vi "Main Tclk.vi"() -> ()   [LabVIEW 2018] (continued)
      n253 = property on="13nA Condenser (V)" class="DigNum (strict)"("Visible"=w181) -> ()  [unwired: 2 in, 2 out]
      n254 = local write "Status message"("standby" ("Status message")) -> ()
      n255 = local write "SEM Options"(w283) -> ()
      n256 = And(x=w164, y=w163) -> (x .and. y?=w162:bool)
      n257 = local write "Reheat completed"(w99) -> ()
      n258 = property on="Status Tabs" class="TabCtl (strict)"() -> ("Pages"=w189:refnum<vi>[])  [unwired: 2 in, 2 out]
      n259 = local write "Unfreeze"(w99) -> ()
      n260 = local write "Scan xn"(w99) -> ()
      n261 = Square Root(x=sgl 2.0 ("t")) -> (sqrt(x)=w104:sgl)
      n262 = local write "Milling para"(w301) -> ()
      n263 = property on="27nA Condenser (V)" class="DigNum (strict)"("Visible"=w181) -> ()  [unwired: 2 in, 2 out]
      n264 = property on="Reheat Output" class="Clust (strict)"("Visible"=w188) -> ()  [unwired: 2 in, 2 out]
      n265 = property on="Turn off FIB gun" class="Bool (strict)"("Visible"=w101) -> ()  [unwired: 2 in, 2 out]
      n266 = property on="Suppressor (V)" class="DigNum (strict)"("Visible"=TRUE) -> ()  [unwired: 2 in, 2 out]
      n267 = Divide(x=w105, y=w104) -> (x/y=w106:sgl)
      n268 = Index Array(array=w189, index=T11."HV Data" ("Status Tabs")) -> (element=w190:refnum<vi>)
      n269 = Select(t=w105, s=w162, f=w106) -> (s? t:f=w161:sgl)
      "X full scale (V)" <- w161
      n270 = local read "File Information"() -> (w286:T31)
      n271 = property class="DAQmx Device"("Active Device"=w248) -> (error out=w242:errorcluster, "AI.PhysicalChans"=w247:tag[])  [unwired: 2 in, 1 out]
      "Logging Channels" <- w247
      n272 = property class="Page"(reference=w190, "PageEnb"=w127) -> ()  [unwired: 1 in, 2 out]
      n273 = shared-variable ".\\Zeiss Library.lvlib\\X full scale (V)"(w161) -> ()  [unwired: 1 in, 1 out]
      n274 = property on="Open FIB gun valve" class="Bool (strict)"("Visible"=w101) -> ()  [unwired: 2 in, 2 out]
      n275 = property on="Image Tabs" class="TabCtl (strict)"() -> ("Pages"=w129:refnum<vi>[])  [unwired: 2 in, 2 out]
      n276 = Bundle By Name(cluster=w286, "File path"=path "E:/Images", "Save recipe"=w110, "Load recipe"=w110) -> (w285:T31)
      n277 = property on="Cursor Z (V)" class="DigNum (strict)"("Visible"=w110) -> ()  [unwired: 2 in, 2 out]
      n278 = Unbundle By Name(w242) -> ("status"=w241:bool)
      n279 = Array Size(array="Parameter Names") -> (size(s)=w244:i32)
      n280 = shared-variable ".\\Zeiss Library.lvlib\\Upload flags path"("D:\\UploadFlags" ("string")) -> ()  [unwired: 1 in, 1 out]
      n281 = property on="FIB Gun Valve Status" class="Str"("Visible"=w101) -> ()  [unwired: 2 in, 2 out]
      n282 = Array Subset(array=w247, length=w244) -> (w246:tag[])  [unwired: 1 in]
      n283 = Index Array(array=w129, index=T37."FIB HV Data" ("Image Tabs")) -> (element=w128:refnum<vi>)
      n284 = Build Path(base path=w113, name or relative path="Email Log") -> (appended path=w197:path)
      "Email Log Files" <- w197
      n285 = Build Path(base path=w113, name or relative path="FIB HV DataLog") -> (appended path=w201:path)
      "FIB HV DataLog Files" <- w201
      n286 = Build Path(base path=w113, name or relative path="SEM HV DataLog") -> (appended path=w152:path)
      "SEM HV DataLog Files" <- w152
      n287 = Build Path(base path=w113, name or relative path="Current DataLog") -> (appended path=w149:path)
      "Current DataLog Files" <- w149
      n288 = Build Path(base path=w113, name or relative path="FIB Reheat Log") -> (appended path=w179:path)
      "FIB Reheat Log Files" <- w179
      n289 = Build Path(base path=w113, name or relative path="Re-engage") -> (appended path=w115:path)
      "Re-engage Files" <- w115
      n290 = Build Path(base path=w113, name or relative path="FIB Probes.csv") -> (appended path=w116:path)
      n291 = Build Path(base path=w113, name or relative path="Last FIB milling snapshot.xml") -> (appended path=→"Last milling snapshot":path)
      n292 = Build Path(base path=w113, name or relative path="Last FIB recipe.csv") -> (appended path=→"Last FIB recipe":path)
      n293 = Build Path(base path=w113, name or relative path="Last FIB image.png") -> (appended path=→"Last FIB image":path)
      n294 = Build Path(base path=w113, name or relative path="Last FIB zoom pre image.png") -> (appended path=→"Last FIB zoom pre image":path)
      n295 = Build Path(base path=w113, name or relative path="Last DetA LM image.png") -> (appended path=→"Last Det A Low Mag":path)
      n296 = Build Path(base path=w113, name or relative path="Last DetB LM image.png") -> (appended path=→"Last Det B Low Mag":path)
      n297 = Build Path(base path=w113, name or relative path="Email alert recipients.txt") -> (appended path=w208:path)
      "Email recipents file" <- w208
      n298 = local write "File Information"(w285) -> ()
      n299 = property class="Page"(reference=w128, "PageEnb"=w127) -> ()  [unwired: 1 in, 2 out]
      n300 = property on="FIB Milling Objective (V)" class="DigNum (strict)"("Visible"=w101) -> ()  [unwired: 2 in, 2 out]
      n301 = property on="FIB Milling Probe" class="CmbBox"("Visible"=w101) -> ()  [unwired: 2 in, 2 out]
      n302 = Path To String(path=w113) -> (string=w114:string)
      n303 = File/Directory Info(path=w197) -> (path out=w194:path, error out=w196:errorcluster)  [unwired: 1 in, 5 out]
      n304 = File/Directory Info(path=w201) -> (path out=w204:path, error out=w202:errorcluster)  [unwired: 1 in, 5 out]
      n305 = File/Directory Info(path=w152) -> (path out=w153:path, error out=w155:errorcluster)  [unwired: 1 in, 5 out]
      n306 = File/Directory Info(path=w149) -> (path out=w148:path, error out=w146:errorcluster)  [unwired: 1 in, 5 out]
      n307 = File/Directory Info(path=w179) -> (path out=w176:path, error out=w178:errorcluster)  [unwired: 1 in, 5 out]
      n308 = File/Directory Info(path=w113) -> (path out=w237:path, error out=w239:errorcluster)  [unwired: 1 in, 5 out]
      n309 = File/Directory Info(path=w115) -> (path out=w218:path, error out=w216:errorcluster)  [unwired: 1 in, 5 out]
      n310 = call-poly <vilib>:"Read Delimited Spreadsheet.vi"("file path (dialog if empty)"=w116, "delimiter (\\t)"="," ("delimiter (\\t)")) -> ("all rows"=w94:string[][])  [unwired: 8 in, 5 out]
      n311 = call <vilib>:"DAQmx Flatten Channel String.vi"("names in"=w246) -> ("names out"=→"Active logging channels":string)  [unwired: 13 in, 1 out]
      n312 = shared-variable ".\\Zeiss Library.lvlib\\3D FIB-SEM Files Path"(w114) -> ()  [unwired: 1 in, 1 out]
      n313 = File/Directory Info(path=w208) -> (path out=w205:path, error out=w207:errorcluster)  [unwired: 1 in, 5 out]
      n314 = Unbundle By Name(w196) -> ("status"=w195:bool)
      n315 = Unbundle By Name(w202) -> ("status"=w203:bool)
      n316 = Unbundle By Name(w178) -> ("status"=w177:bool)
      n317 = Unbundle By Name(w216) -> ("status"=w217:bool)
      n318 = Array Size(array=w94) -> (size(s)=w122:i32[])
      n319 = Unbundle By Name(w155) -> ("status"=w154:bool)
      n320 = Unbundle By Name(w146) -> ("status"=w147:bool)
      n321 = Unbundle By Name(w239) -> ("status"=w238:bool)
      n322 = property on="Min FIB probe" class="Bool (strict)"("Visible"=w101) -> ()  [unwired: 2 in, 2 out]
      n323 = property on="Save Probe Table" class="Bool (strict)"("Visible"=w101) -> ()  [unwired: 2 in, 2 out]
      n324 = Unbundle By Name(w207) -> ("status"=w206:bool)
      n325 = Index Array(array=w122, index=0) -> (element=w121:i32)
      n326 = Decrement(x=w121) -> (x-1=w124:i32)
      n327 = case shown="True" w195 {
        tunnel: w194 -> [_ w435]
        frame False {
        }
        frame True {
          n328 = Create Folder(path (use dialog)=w435) -> ()  [unwired: 1 in, 4 out]
        }
      }
      n329 = case shown="True" w203 {
        tunnel: w204 -> [_ w436]
        frame False {
        }
        frame True {
          n330 = Create Folder(path (use dialog)=w436) -> ()  [unwired: 1 in, 4 out]
        }
      }
      n331 = case shown="True" w154 {
        tunnel: w153 -> [_ w322]
        frame False {
        }
        frame True {
          n332 = Create Folder(path (use dialog)=w322) -> ()  [unwired: 1 in, 4 out]
        }
      }
      n333 = case shown="True" w147 {
        tunnel: w148 -> [_ w321]
        frame False {
        }
        frame True {
          n334 = Create Folder(path (use dialog)=w321) -> ()  [unwired: 1 in, 4 out]
        }
      }
      n335 = case shown="True" w177 {
        tunnel: w176 -> [_ w434]
        frame False {
        }
        frame True {
          n336 = Create Folder(path (use dialog)=w434) -> ()  [unwired: 1 in, 4 out]
        }
      }
      n337 = case shown="True" w238 {
        tunnel: w237 -> [_ w459]
        frame False {
        }
        frame True {
          n338 = Create Folder(path (use dialog)=w459) -> ()  [unwired: 1 in, 4 out]
        }
      }
      n339 = case shown="True" w217 {
        tunnel: w218 -> [_ w458]
        frame False {
        }
        frame True {
          n340 = Create Folder(path (use dialog)=w458) -> ()  [unwired: 1 in, 4 out]
        }
      }
      n341 = property on="Image Tabs" class="TabCtl (strict)"() -> ("Pages"=w186:refnum<vi>[])  [unwired: 2 in, 2 out]
      n342 = property on="Max FIB probe" class="Bool (strict)"("Visible"=w101) -> ()  [unwired: 2 in, 2 out]
      n343 = Index Array(array=w94, index (row)=w124) -> (element=w119:string[])  [unwired: 1 in]
      n344 = case shown="False" w206 {
        tunnel: w205 -> [w444 _]
        frame False {
          n345 = Open/Create/Replace File(file path (use dialog)=w444) -> (refnum out=w445:refnum<file>, error out=w446:errorcluster)  [unwired: 5 in, 1 out]
          n346 = local read "Mail server"() -> (w441:string)
          n347 = local read "Hardware Configuration"() -> (w439:T25)
          n348 = Read from Text File(file (use dialog)=w445, error in=w446) -> (refnum out=w447:refnum<file>, text=w443:string, error out=w448:errorcluster)  [unwired: 2 in, 1 out]
          n349 = while {
            shift-right: [w456] -> _
            shift-left: w443 -> [w453]
            tunnel: [w455] -> w437 mode=indexing
            stop <- w449 stop-if-true
            n350 = String Length(string=w453) -> (length=w452:i32)
            n351 = Match Pattern(string=w453, regular expression="\n") -> (before substring=w455:string, after substring=w456:string, offset past match=w454:i32)  [unwired: 1 in, 1 out]
            n352 = local read "Off"() -> (w450:bool)
            n353 = Equal?(x=w454, y=w452) -> (x = y?=w451:bool)
            n354 = Or(x=w451, y=w450) -> (x .or. y?=w449:bool)
          }
          n355 = Close File(refnum=w447, error in=w448) -> ()  [unwired: 2 out]
          n356 = Unbundle By Name(w439) -> ("Machine ID"=w440:string)
          n357 = local write "Email Alert Recipients"(w437) -> ()
          n358 = call "Email alert.vi"("Send email"=TRUE, "Machine ID"=w440, "Mail server"=w441, "Alarm message"="3D FIB-SEM restarted", "Recipents"=w437) -> ()  [unwired: 7 in]
        }
        frame True {
        }
      }
      n359 = Delete From Array(array=w119, length=1, index=0) -> (array with subset deleted=w108:string[])  [unwired: 1 out]
      n360 = case shown="False" w241 {
        frame False {
          w460 = TRUE ("Enable logging")
          n361 = local write "Enable logging"(TRUE ("Enable logging")) -> ()
          n362 = property on="Sample rate (Hz)" class="DigNum (strict)"("Visible"=w460) -> ()  [unwired: 2 in, 2 out]
          n363 = property on="Samples size" class="DigNum (strict)"("Visible"=w460) -> ()  [unwired: 2 in, 2 out]
          n364 = property on="Logging Channels" class="Arr (strict)"("Visible"=w460) -> ()  [unwired: 2 in, 2 out]
          n365 = property on="Parameter Names" class="Arr (strict)"("Visible"=w460) -> ()  [unwired: 2 in, 2 out]
          n366 = property on="Measurements" class="WFChart (strict)"("Visible"=w460) -> ()  [unwired: 2 in, 2 out]
          n367 = property on="Clear" class="Bool"("Visible"=w460) -> ()  [unwired: 2 in, 2 out]
          n368 = property on="Enable logging" class="Bool (strict)"("DisabledEnum"=T44."Enabled" ("Disabled")) -> ()  [unwired: 2 in, 2 out]
        }
        frame True {
          w463 = FALSE ("Enable logging")
          n369 = local write "Enable logging"(FALSE ("Enable logging")) -> ()
          n370 = property on="Sample rate (Hz)" class="DigNum (strict)"("Visible"=w463) -> ()  [unwired: 2 in, 2 out]
          n371 = property on="Samples size" class="DigNum (strict)"("Visible"=w463) -> ()  [unwired: 2 in, 2 out]
          n372 = property on="Logging Channels" class="Arr (strict)"("Visible"=w463) -> ()  [unwired: 2 in, 2 out]
          n373 = property on="Parameter Names" class="Arr (strict)"("Visible"=w463) -> ()  [unwired: 2 in, 2 out]
          n374 = property on="Measurements" class="WFChart (strict)"("Visible"=w463) -> ()  [unwired: 2 in, 2 out]
          n375 = property on="Clear" class="Bool"("Visible"=w463) -> ()  [unwired: 2 in, 2 out]
          n376 = property on="Enable logging" class="Bool (strict)"("DisabledEnum"=T44."Disabled and Grayed Out" ("Disabled")) -> ()  [unwired: 2 in, 2 out]
        }
      }
      n377 = property on="FIB probe switching" class="Str"("Visible"=w101) -> ()  [unwired: 2 in, 2 out]
      n378 = Index Array(array=w186, index=T37."FIB Milling Offset after Pause" ("Image Tabs")) -> (element=w185:refnum<vi>)
      n379 = Build Cluster Array(w108, w108) -> (w98:cluster{"String":string, "String":string}[])
      n380 = property class="Page"(reference=w185, "PageVis"=FALSE ("Page Visible")) -> ()  [unwired: 1 in, 2 out]
      n381 = local read "FIB Scan Parameters"() -> (w135:T32)
      n382 = property on="FIB Milling Probe" class="CmbBox"("Strings And Values[]"=w98) -> ()  [unwired: 2 in, 2 out]
      n383 = shared-variable "My Computer\\Zeiss Library.lvlib\\FIB Probes"(w108) -> ()  [unwired: 1 in, 1 out]
      n384 = local read "Milling para"() -> (w143:T35)
      n385 = control-ref of="FIB Image"() -> (w144:refnum<vi>)
      n386 = local read "FIB Scan Parameters"() -> (w142:T32)
      n387 = local read "FIB Options"() -> (w141:T33)
      n388 = shared-variable ".\\Zeiss Library.lvlib\\Milling Z Voltage RT"() -> (w139:sgl)  [unwired: 1 in, 1 out]
      n389 = property on="FIB HV target matched" class="Bool (strict)"("Visible"=w101) -> ()  [unwired: 2 in, 2 out]
      n390 = property on="Get V/I slope" class="Bool (strict)"("Visible"=w101) -> ()  [unwired: 2 in, 2 out]
      n391 = Unbundle By Name(w135) -> ("Z resolution"=w134:u32, "X resolution"=w133:u32)
      n392 = property on="FIB Imaging Probe" class="CmbBox"("Strings And Values[]"=w98) -> ()  [unwired: 2 in, 2 out]
      n393 = property on="FIB probe auto min" class="Bool (strict)"("Visible"=w101) -> ()  [unwired: 2 in, 2 out]
      n394 = property on="FIB V/I slope" class="DigNum (strict)"("Visible"=w101) -> ()  [unwired: 2 in, 2 out]
      n395 = call "FIB image draw milling.vi"("Milling Z Voltage"=w139, "Milling para"=w143, "FIB Options"=w141, "FIB Scan Parameters"=w142, "Origin"=TRUE, "Image reference"=w144) -> ("Trapezoidal"=w138:cluster{"X":i16, "Y":i16}[])  [unwired: 4 in, 1 out]
      n396 = Initialize Array(i16 0 ("element"), w134, w133) -> (w137:i16[][])
      n397 = local write "Trapezoidal"(w138) -> ()
      n398 = local write "FIB Image"(w137) -> ()
      n399 = property on="Mill start from Last" class="Bool (strict)"("DisabledEnum"=w103) -> ()  [unwired: 2 in, 2 out]
      n400 = property on="Scan x1" class="Bool (strict)"("DisabledEnum"=w103) -> ()  [unwired: 2 in, 2 out]
      n401 = property on="Scan xn" class="Bool (strict)"("DisabledEnum"=w103) -> ()  [unwired: 2 in, 2 out]
      n402 = property on="FIB Imaging" class="Bool (strict)"("DisabledEnum"=w103) -> ()  [unwired: 2 in, 2 out]
      n403 = property on="FIB time lapse" class="Bool (strict)"("DisabledEnum"=w103) -> ()  [unwired: 2 in, 2 out]
      n404 = property on="Reset" class="Bool (strict)"("DisabledEnum"=w103) -> ()  [unwired: 2 in, 2 out]
      n405 = property on="Pre image" class="Bool (strict)"("DisabledEnum"=w103) -> ()  [unwired: 2 in, 2 out]
      n406 = property on="Post image" class="Bool (strict)"("DisabledEnum"=w103) -> ()  [unwired: 2 in, 2 out]
      n407 = property on="Mill" class="Bool (strict)"("DisabledEnum"=w103) -> ()  [unwired: 2 in, 2 out]
      n408 = property on="Mill Manual Pause" class="Bool (strict)"("DisabledEnum"=w103) -> ()  [unwired: 2 in, 2 out]
      n409 = property on="Z-step (nm)" class="DigNum (strict)"("DisabledEnum"=w103) -> ()  [unwired: 2 in, 2 out]
      n410 = property on="X min index" class="DigNum (strict)"("Visible"=w222) -> ()  [unwired: 2 in, 2 out]
      n411 = property on="X max index" class="DigNum (strict)"("Visible"=w222) -> ()  [unwired: 2 in, 2 out]
      n412 = property on="AF Steps" class="DigNum (strict)"("DisabledEnum"=w103) -> ()  [unwired: 2 in, 2 out]
      n413 = property on="AS Steps" class="DigNum (strict)"("DisabledEnum"=w103) -> ()  [unwired: 2 in, 2 out]
      n414 = property on="AA Steps" class="DigNum (strict)"("DisabledEnum"=w103) -> ()  [unwired: 2 in, 2 out]
      n415 = property on="Start Current DataLog" class="Bool (strict)"("DisabledEnum"=w103) -> ()  [unwired: 2 in, 2 out]
      n416 = property on="Detector C name" class="Str"("DisabledEnum"=w199) -> ()  [unwired: 2 in, 2 out]
      n417 = property on="Detector D name" class="Str"("DisabledEnum"=w199) -> ()  [unwired: 2 in, 2 out]
      n418 = property on="Pause for reheat" class="Bool (strict)"("DisabledEnum"=w199) -> ()  [unwired: 2 in, 2 out]
      n419 = property on="Request to stop reheat" class="Bool (strict)"("DisabledEnum"=w199) -> ()  [unwired: 2 in, 2 out]
      "3D FIB-SEM Files" <- w113
      "Reheat complete file" <- path "C:/Program Files (x86)/FEI Company/BDS/Reheat/Complete.txt" ("Log file path")
      "Reheat stopped file" <- path "C:/Program Files (x86)/FEI Company/BDS/Reheat/Stopped.txt" ("Log file path")
      "FIB emission below limit counts" <- w97
      "FI below limit counts" <- w97
      "WD array tiled" <- w172
      "ASX Success tiled" <- w96
      "ASY Success tiled" <- w96
      "AAY Success tiled" <- w96
      "AF Success tiled" <- w96
      "FI array" <- w95
      "FI grid array" <- w172
      "FI array tiled" <- w172
      "FI grid array tiled" <- sgl[][][][][] [] ("FI grid array tiled")
      "Best WD FI tiled" <- w174
      "Best WD (mm) tiled" <- w174
      "Slope tiled" <- w174
      "StigX array tiled" <- w172
      "Best Stig X FI tiled" <- w174
      "Best Stig X (%) tiled" <- w174
      "StigY array tiled" <- w172
      "AlnX array tiled" <- w172
      "AlnY array tiled" <- w172
      "Best Stig Y FI tiled" <- w174
      "Best Stig Y (%) tiled" <- w174
      "Best Aln X FI tiled" <- w174
      "Best Aln X (%) tiled" <- w174
      "Best Aln Y FI tiled" <- w174
      "Best Aln Y (%) tiled" <- w174
      "Skip Steps tiled" <- u8[][] [] ("FI array")
      "FIB CL I out of bound counts" <- w97
      "AF Count" <- w97
      "AS Count" <- w97
      "AA Count" <- w97
      "WD Stig Aln tile offsets" <- T42 {[], [], [], [], [], [], []} ("output cluster")
      "Reheat start file" <- path "C:/Program Files (x86)/FEI Company/BDS/Reheat/Start.txt" ("Log file path")
      "Milling mode" <- T10."FIB" ("FIB mode")
      "LM overhead" <- w97
      "MM overhead" <- w97
      "Re-engage counts" <- w97
      "Recovered counts" <- w97
      "Last re-engage count" <- w97
      "FIB slice #" <- w97
      "3D image paused active" <- w99
      "FIB probe switching" <- "Go to                 or               current of the same probe " ("FIB probe switching")
      "FIB suppressor below limit counts" <- w97
      "Continued fine milling frames" <- w97
      "Specimen I out of bound" <- w99
      "BD2 out of bound" <- w99
      "Milling I out of bound" <- w99
      "BD1 out of bound" <- w99
      "API timeout" <- w99
      "Remaining Y shift frames" <- w97
      "Remaining X shift frames" <- w97
      "AAX Success tiled" <- w96
    }
    frame #2 {
      n420 = flat-sequence {
        frame #0 {
          w677 = u16 2 items=["Operate", "Initialize", "Read from .INI", "Write to .INI"] ("Action")
          w679 = u16 1 items=["Operate", "Initialize", "Read from .INI", "Write to .INI"] ("Action")
          n421 = local read "Hardware Configuration"() -> (w680:T25)
          n422 = Unbundle By Name(w680) -> ("Configuration file"=w675:path, "Shutter Drive"=w676:tag)
          n423 = call "Shutter Core with Damping Option V2.vi"("Shutter Drive"=w676, "Action"=w679, "path to .INI file"=w675) -> ("file path Out"=w678:path)  [unwired: 5 in, 3 out]
          n424 = call "Shutter Core with Damping Option V2.vi"("Shutter Drive"=w676, "Action"=w677, "path to .INI file"=w678) -> ()  [unwired: 5 in, 4 out]
        }
        frame #1 {
          n425 = local read "Hardware Configuration"() -> (w689:T25)
          n426 = local read "Damping"() -> (w682:bool)
          n427 = Unbundle By Name(w689) -> ("Shutter Drive"=w688:tag)
          n428 = call "Shutter Swing V3.vi"("Retry #"=1, "Shutter Drive"=w688, "Damping"=w682, "Shutter close"=TRUE) -> ("Shutter close fdbk"=w683:bool, "Fail #"=w684:u8, "SEM shutter status"=w685:string, "Color Box"=w686:u32)  [unwired: 1 in, 3 out]
          n429 = property on="SEM shutter status" class="Str"("Text.BGColor"=w686) -> ()  [unwired: 2 in, 2 out]
          n430 = local write "SEM shutter status"(w685) -> ()
          n431 = local write "Fail #"(w684) -> ()
          n432 = local write "SEM Shutter"(w683) -> ()
        }
        frame #2 {
          w690 = u16 1 items=["Do Nothing", "Send Idle Only", "Watch FIB & SEM", "Watch FIB Only", "Watch SEM Only"] ("WatchDog Mode")
          # "Put Watchdog into Idle mode"
          n433 = call "FM Gen Pulse for FIB-SEM.vi"("WatchDog Mode"=w690, "State Value"=i16 1) -> ()  [unwired: 7 in, 3 out]
        }
        frame #3 {
          w695 = -10.0 ("Output voltage (V)")
          n434 = local read "Hardware Configuration"() -> (w693:T25)
          n435 = Unbundle By Name(w693) -> ("SEM X coil"=w692:refnum<k15>, "SEM Y coil"=w694:refnum<k15>)
          n436 = call "FGEN DC voltage.vi"("Output voltage (V)"=w695, "Resource Name"=w692) -> ()  [unwired: 9 in, 1 out]
          n437 = call "FGEN DC voltage.vi"("Output voltage (V)"=w695, "Resource Name"=w694) -> ()  [unwired: 9 in, 1 out]
        }
        frame #4 {
          n438 = local read "Hardware Configuration"() -> (w704:T25)
          n439 = local read "Damping"() -> (w698:bool)
          n440 = Unbundle By Name(w704) -> ("Shutter Drive"=w703:tag)
          n441 = call "Shutter Swing V3.vi"("Retry #"=1, "Shutter Drive"=w703, "Damping"=w698, "Shutter close"=FALSE) -> ("Shutter close fdbk"=w699:bool, "Fail #"=w696:u8, "SEM shutter status"=w700:string, "Color Box"=w701:u32)  [unwired: 1 in, 3 out]
          n442 = property on="SEM shutter status" class="Str"("Text.BGColor"=w701) -> ()  [unwired: 2 in, 2 out]
          n443 = local write "SEM shutter status"(w700) -> ()
          n444 = local write "Fail #"(w696) -> ()
          n445 = local write "SEM Shutter"(w699) -> ()
        }
        frame #5 {
          n446 = local write "Fail #"(u8 0 ("Fail #")) -> ()
        }
      }
    }
    frame #3 {
      w707 = u32 0 ("FIB slice #")
      # "Sends out a \"heartbeat\" signal to watchdog.\nIf watchdog is in an active monitoring state (2-5)\nand does not get this state a few times (default 5)\nin a row, it will go to \"protect\" and close the gate valves.\nProtects against \"3D FIB-SEM.exe\" locking up and leaving\nPXIe box stuck scanning SEM even if we are not including\n\"monitor SEM\" in \"watchdog mode\""
      n447 = Current VI's Path() -> (path=w709:path)
      n448 = while {
        stop <- w5784 stop-if-true
        n449 = stacked-sequence {
          tunnel: [_ w5812] -> w5784
          frame #0 {
            n450 = local read "Unfreeze"() -> (w5786:bool)
            n451 = case shown="True" w5786 {
              frame False {
              }
              frame True {
                n452 = stacked-sequence {
                  frame #0 {
                    w5788 = T44."Disabled and Grayed Out" ("Disabled")
                    n453 = local read "FIB HW Config"() -> (w5794:T23)
                    n454 = local read "FIB HW Config"() -> (w5791:T23)
                    n455 = local read "Api"() -> (w5787:refnum<k7>)
                    n456 = Unbundle By Name(w5794) -> ("Beam blank"=w5793:tag)
                    n457 = Unbundle By Name(w5791) -> ("FIB Ext Scan"=w5789:tag)
                    n458 = call "FIB beam blank.vi"("ActiveX Container"=w5787, "Beam blanked"=TRUE, "lines"=w5793) -> ()  [unwired: 2 in, 1 out]
                    n459 = call "FIB ext scan.vi"("Ext on"=TRUE ("data"), "FIB Ext Scan"=w5789) -> ()  [unwired: 9 in, 1 out]
                    n460 = property on="Pre image" class="Bool (strict)"("DisabledEnum"=w5788) -> ()  [unwired: 2 in, 2 out]
                    n461 = property on="Post image" class="Bool (strict)"("DisabledEnum"=w5788) -> ()  [unwired: 2 in, 2 out]
                  }
                  frame #1 {
                    n462 = local read "COM port"() -> (w5797:refnum<visa-resource-name>)
                    n463 = local read "FIB HW Config"() -> (w5798:T23)
                    n464 = local read "FIB Options"() -> (w5801:T33)
                    n465 = local read "FIB single scan"() -> (w5796:bool)
                    n466 = local read "FIB Scan Parameters"() -> (w5802:T32)
                    n467 = local read "Api"() -> (w5795:refnum<k7>)
                    n468 = call "FIB realtime imaging PXIe-6124.vi"("HW Config"=w5798, "Options"=w5801, "Single scan"=w5796, "Scan Para"=w5802, "As subVi"=TRUE, "COM port"=w5797, "ActiveX Container"=w5795) -> ("error out"=w5800:errorcluster)  [unwired: 2 in, 1 out]
                    n469 = Unbundle By Name(w5801) -> ("Scan mode"=w5803:u16)
                    n470 = Unbundle By Name(w5802) -> ("X resolution"=w5805:u32, "Z resolution"=w5804:u32)
                    n471 = Unbundle By Name(w5800) -> ("status"=w5799:bool)
                    n472 = Equal To 0?(x=w5803) -> (x = 0?=w5807:bool)
                    n473 = Bundle("X resolution"=w5805, "Z resolution"=w5804) -> (w5806:cluster{"X resolution":u32, "Z resolution":u32})  [unwired: 1 in]
                    n474 = property on="X resolution with rampdown" class="DigNum (strict)"("Visible"=w5807) -> ()  [unwired: 2 in, 2 out]
                    n475 = case shown="True" w5799 {
                      frame False {
                      }
                      frame True {
                        n476 = local write "Unfreeze"(FALSE ("Freeze")) -> ()
                      }
                    }
                    n477 = property on="FIB Image" class="IntGraph (strict)"("Plot Area Size"=w5806) -> ()  [unwired: 2 in, 2 out]
                  }
                  frame #2 {
                    n478 = local read "FIB single scan"() -> (w5810:bool)
                    n479 = case shown="True" w5810 {
                      frame False {
                      }
                      frame True {
                        w5811 = FALSE ("FIB single scan")
                        n480 = local write "FIB single scan"(w5811) -> ()
                        n481 = local write "FIB Imaging"(w5811) -> ()
                        n482 = local write "Unfreeze"(w5811) -> ()
                      }
                    }
                  }
                }
              }
            }
          }
          frame #1 {
            n483 = local read "Stop"() -> (w5812:bool)
            n484 = case shown="True" w5812 {
              frame False {
              }
              frame True {
                n485 = local read "FIB HW Config"() -> (w5816:T23)
                n486 = Unbundle By Name(w5816) -> ("Beam blank"=w5815:tag)
                n487 = local read "Api"() -> (w5813:refnum<k7>)
                n488 = call "FIB beam blank.vi"("ActiveX Container"=w5813, "Beam blanked"=TRUE, "lines"=w5815) -> ()  [unwired: 2 in, 1 out]
              }
            }
          }
        }
        n489 = Wait Until Next ms Multiple(millisecond multiple=u32 100) -> ()  [unwired: 1 out]
      }
      n490 = while {
        stop <- w5818 stop-if-true
        n491 = case shown="True" "FIB" {
          tunnel: [w5830 w5838] -> w5818
          frame False {
            w5822 = u8 0 ("AF Count")
            w5825 = sgl[][][] [] ("FI grid array")
            w5826 = FALSE ("Rect Milling Line Paused")
            w5820 = T44."Enabled" ("Disabled")
            n492 = local write "AF Count"(w5822) -> ()
            n493 = local write "AS Count"(w5822) -> ()
            n494 = local write "AA Count"(w5822) -> ()
            n495 = local write "Skip Steps tiled"(u8[][] [] ("Skip Steps tiled")) -> ()
            n496 = local write "Stig Options"(enum16{"Defaut", "Stig X", "Stig Y"}."Defaut" ("Stig Options")) -> ()
            n497 = local write "Auto Focus"(w5826) -> ()
            n498 = local write "Auto Stig"(w5826) -> ()
            n499 = local write "Auto Align"(w5826) -> ()
            n500 = local write "Mill Manual Pause"(w5826) -> ()
            n501 = local write "Mill Stop"(w5826) -> ()
            n502 = local write "Pause for reheat"(w5826) -> ()
            n503 = local read "Stop"() -> (w5830:bool)
            n504 = local write "FI grid array"(w5825) -> ()
            n505 = local write "FI array tiled"(w5825) -> ()
            n506 = local write "WD array tiled"(w5825) -> ()
            n507 = local write "StigX array tiled"(w5825) -> ()
            n508 = local write "StigY array tiled"(w5825) -> ()
            n509 = local write "AlnX array tiled"(w5825) -> ()
            n510 = local write "AlnY array tiled"(w5825) -> ()
            n511 = shared-variable "My Computer\\Zeiss Library.lvlib\\Milling Stop"(w5830) -> ()  [unwired: 1 in, 1 out]
            n512 = local write "Aln Options"(enum16{"Defaut", "Aln X", "Aln Y"}."Defaut" ("Aln Options")) -> ()
            n513 = property on="Mill start from Last" class="Bool (strict)"("DisabledEnum"=w5820) -> ()  [unwired: 2 in, 2 out]
            n514 = property on="Keep aspect ratio" class="Bool (strict)"("DisabledEnum"=w5820) -> ()  [unwired: 2 in, 2 out]
            n515 = property on="X Grids" class="Arr (strict)"("DisabledEnum"=w5820) -> ()  [unwired: 2 in, 2 out]
            n516 = property on="Y Grids" class="Arr (strict)"("DisabledEnum"=w5820) -> ()  [unwired: 2 in, 2 out]
            n517 = property on="Primary X index" class="Arr (strict)"("DisabledEnum"=w5820) -> ()  [unwired: 2 in, 2 out]
            n518 = property on="Primary Y index" class="Arr (strict)"("DisabledEnum"=w5820) -> ()  [unwired: 2 in, 2 out]
            n519 = property on="Scan x1" class="Bool (strict)"("DisabledEnum"=w5820) -> ()  [unwired: 2 in, 2 out]
            n520 = property on="Scan xn" class="Bool (strict)"("DisabledEnum"=w5820) -> ()  [unwired: 2 in, 2 out]
            n521 = property on="FIB Imaging" class="Bool (strict)"("DisabledEnum"=w5820) -> ()  [unwired: 2 in, 2 out]
            n522 = property on="FIB time lapse" class="Bool (strict)"("DisabledEnum"=w5820) -> ()  [unwired: 2 in, 2 out]
            n523 = property on="Auto Focus" class="Bool (strict)"("DisabledEnum"=w5820) -> ()  [unwired: 2 in, 2 out]
            n524 = property on="Auto Stig" class="Bool (strict)"("DisabledEnum"=w5820) -> ()  [unwired: 2 in, 2 out]
            n525 = property on="Auto Align" class="Bool (strict)"("DisabledEnum"=w5820) -> ()  [unwired: 2 in, 2 out]
            n526 = property on="Reset" class="Bool (strict)"("DisabledEnum"=w5820) -> ()  [unwired: 2 in, 2 out]
            n527 = property on="AF Steps" class="DigNum (strict)"("DisabledEnum"=w5820) -> ()  [unwired: 2 in, 2 out]
            n528 = property on="AS Steps" class="DigNum (strict)"("DisabledEnum"=w5820) -> ()  [unwired: 2 in, 2 out]
            n529 = property on="AA Steps" class="DigNum (strict)"("DisabledEnum"=w5820) -> ()  [unwired: 2 in, 2 out]
            n530 = property on="Beam blanked" class="Bool (strict)"("DisabledEnum"=w5820) -> ()  [unwired: 2 in, 2 out]
            n531 = property on="Spot" class="Bool (strict)"("DisabledEnum"=w5820) -> ()  [unwired: 2 in, 2 out]
            n532 = property on="Mill Stop" class="Bool (strict)"("DisabledEnum"=w5820) -> ()  [unwired: 2 in, 2 out]
            n533 = property on="ROI" class="Bool (strict)"("DisabledEnum"=w5820) -> ()  [unwired: 2 in, 2 out]
            n534 = property on="FIB Profile" class="Bool (strict)"("DisabledEnum"=w5820) -> ()  [unwired: 2 in, 2 out]
            n535 = property on="FIB FOV (um)" class="DigNum (strict)"("DisabledEnum"=w5820) -> ()  [unwired: 2 in, 2 out]
            n536 = property on="X center (um)" class="DigNum (strict)"("DisabledEnum"=w5820) -> ()  [unwired: 2 in, 2 out]
            n537 = property on="Z center (um)" class="DigNum (strict)"("DisabledEnum"=w5820) -> ()  [unwired: 2 in, 2 out]
            n538 = property on="X size (um)" class="DigNum (strict)"("DisabledEnum"=w5820) -> ()  [unwired: 2 in, 2 out]
            n539 = property on="Z size (um)" class="DigNum (strict)"("DisabledEnum"=w5820) -> ()  [unwired: 2 in, 2 out]
            n540 = property on="X resolution" class="DigNum (strict)"("DisabledEnum"=w5820) -> ()  [unwired: 2 in, 2 out]
            n541 = property on="Z resolution" class="DigNum (strict)"("DisabledEnum"=w5820) -> ()  [unwired: 2 in, 2 out]
            n542 = property on="Z-step (nm)" class="DigNum (strict)"("DisabledEnum"=w5820) -> ()  [unwired: 2 in, 2 out]
            n543 = property on="Start Current DataLog" class="Bool (strict)"("DisabledEnum"=w5820) -> ()  [unwired: 2 in, 2 out]
            n544 = local read "Machine Type"() -> (w5821:u8)
            n545 = local read "Unfreeze"() -> (w5828:bool)
            n546 = case shown="2" w5821 {
              frame 0, Default {
              }
              frame 2 {
                n547 = local read "Api"() -> (w5836:refnum<k7>)
                n548 = call "SmartSEM Remote API set float.vi"("vValue"=sgl 0.0, "lpszParam"="DP_PANEL_DISABLE", "ActiveX Container"=w5836) -> ("reference out"=w5832:refnum<k7>)  [unwired: 7 in, 1 out]
                n549 = call "SmartSEM Remote API set float.vi"("vValue"=sgl 0.0, "lpszParam"="DP_JOYSTICK_DISABLE", "ActiveX Container"=w5832) -> ()  [unwired: 7 in, 2 out]
              }
            }
            n550 = case shown="False" w5828 {
              tunnel: w5820 -> [w5837 _]
              frame False {
                n551 = property on="Pre image" class="Bool (strict)"("DisabledEnum"=w5837) -> ()  [unwired: 2 in, 2 out]
                n552 = property on="Post image" class="Bool (strict)"("DisabledEnum"=w5837) -> ()  [unwired: 2 in, 2 out]
                n553 = property on="Mill" class="Bool (strict)"("DisabledEnum"=w5837) -> ()  [unwired: 2 in, 2 out]
                n554 = property on="Mill Manual Pause" class="Bool (strict)"("DisabledEnum"=w5837) -> ()  [unwired: 2 in, 2 out]
              }
              frame True {
              }
            }
            n555 = property on="Pause for reheat" class="Bool (strict)"("DisabledEnum"=T44."Disabled and Grayed Out" ("Disabled")) -> ()  [unwired: 2 in, 2 out]
          }
          frame True {
            n556 = stacked-sequence {
              tunnel: [_ _ _ _ _ _ _ w6166 _ _ _ _ _ _ _ _ _ _ _ _ _ _ _ _ _ _ _ _ _ _ _ _ _ _ _ _ _ _ _ _ _ _ _] -> w5838
              frame #0 {
                w5841 = TRUE ("SW error warning armed")
                w5839 = T44."Disabled and Grayed Out" ("Disabled")
                n557 = local read "FIB HW Config"() -> (w5850:T23)
                n558 = local read "FIB HW Config"() -> (w5853:T23)
                n559 = local read "Api"() -> (w5840:refnum<k7>)
                n560 = Unbundle By Name(w5850) -> ("Beam blank"=w5851:tag)
                n561 = Unbundle By Name(w5853) -> ("FIB Ext Scan"=w5854:tag)
                n562 = local read "Milling para"() -> (w5846:T35)
                n563 = property on="Pause for reheat" class="Bool (strict)"("DisabledEnum"=T44."Enabled" ("Disabled")) -> ()  [unwired: 2 in, 2 out]
                n564 = property on="Scan x1" class="Bool (strict)"("DisabledEnum"=w5839) -> ()  [unwired: 2 in, 2 out]
                n565 = property on="Mill start from Last" class="Bool (strict)"("DisabledEnum"=w5839) -> ()  [unwired: 2 in, 2 out]
                n566 = property on="Scan xn" class="Bool (strict)"("DisabledEnum"=w5839) -> ()  [unwired: 2 in, 2 out]
                n567 = property on="FIB Imaging" class="Bool (strict)"("DisabledEnum"=w5839) -> ()  [unwired: 2 in, 2 out]
                n568 = property on="FIB time lapse" class="Bool (strict)"("DisabledEnum"=w5839) -> ()  [unwired: 2 in, 2 out]
                n569 = property on="Reset" class="Bool (strict)"("DisabledEnum"=w5839) -> ()  [unwired: 2 in, 2 out]
                n570 = property on="Pre image" class="Bool (strict)"("DisabledEnum"=w5839) -> ()  [unwired: 2 in, 2 out]
                n571 = property on="Post image" class="Bool (strict)"("DisabledEnum"=w5839) -> ()  [unwired: 2 in, 2 out]
                n572 = call "FIB ext scan.vi"("Ext on"=TRUE, "FIB Ext Scan"=w5854) -> ()  [unwired: 9 in, 1 out]
                n573 = call "FIB beam blank.vi"("ActiveX Container"=w5840, "Beam blanked"=TRUE, "lines"=w5851) -> ()  [unwired: 2 in, 1 out]
                n574 = Unbundle By Name(w5846) -> ("Mill start from Last"=w5845:bool)
                n575 = property on="Beam blanked" class="Bool (strict)"("DisabledEnum"=w5839) -> ()  [unwired: 2 in, 2 out]
                n576 = property on="FIB Profile" class="Bool (strict)"("DisabledEnum"=w5839) -> ()  [unwired: 2 in, 2 out]
                n577 = property on="Start Current DataLog" class="Bool (strict)"("DisabledEnum"=w5839) -> ()  [unwired: 2 in, 2 out]
                n578 = property on="Spot" class="Bool (strict)"("DisabledEnum"=w5839) -> ()  [unwired: 2 in, 2 out]
                n579 = property on="Mill Stop" class="Bool (strict)"("DisabledEnum"=w5839) -> ()  [unwired: 2 in, 2 out]
                n580 = property on="ROI" class="Bool (strict)"("DisabledEnum"=w5839) -> ()  [unwired: 2 in, 2 out]
                n581 = property on="Mill" class="Bool (strict)"("DisabledEnum"=w5839) -> ()  [unwired: 2 in, 2 out]
                n582 = local read "FIB slice #"() -> (w5849:u32)
                n583 = shared-variable "My Computer\\Zeiss Library.lvlib\\Milling cont. from Last"(w5845) -> ()  [unwired: 1 in, 1 out]
                n584 = local write "SW error warning armed"(w5841) -> ()
                n585 = local write "SEM shutter warning armed"(w5841) -> ()
                n586 = local write "Start Current DataLog"(FALSE ("Start Current DataLog")) -> ()
                n587 = property on="FIB FOV (um)" class="DigNum (strict)"("DisabledEnum"=w5839) -> ()  [unwired: 2 in, 2 out]
                n588 = property on="X center (um)" class="DigNum (strict)"("DisabledEnum"=w5839) -> ()  [unwired: 2 in, 2 out]
                n589 = property on="X resolution" class="DigNum (strict)"("DisabledEnum"=w5839) -> ()  [unwired: 2 in, 2 out]
                n590 = property on="Z resolution" class="DigNum (strict)"("DisabledEnum"=w5839) -> ()  [unwired: 2 in, 2 out]
                n591 = property on="Z-step (nm)" class="DigNum (strict)"("DisabledEnum"=w5839) -> ()  [unwired: 2 in, 2 out]
                n592 = property on="Z center (um)" class="DigNum (strict)"("DisabledEnum"=w5839) -> ()  [unwired: 2 in, 2 out]
                n593 = property on="X size (um)" class="DigNum (strict)"("DisabledEnum"=w5839) -> ()  [unwired: 2 in, 2 out]
                n594 = property on="Z size (um)" class="DigNum (strict)"("DisabledEnum"=w5839) -> ()  [unwired: 2 in, 2 out]
                n595 = Equal To 0?(x=w5849) -> (x = 0?=w5848:bool)
                n596 = And(x=w5848, y=w5845) -> (x .and. y?=w5847:bool)
                n597 = case shown="True" w5847 {
                  frame False {
                    w5855 = u8 0 ("Stage move flag")
                    n598 = local read "Additional Info"() -> (w5857:cluster{"Restart flag":u8, "Stage move flag":u8})
                    n599 = Bundle By Name(cluster=w5857, "Restart flag"=w5855, "Stage move flag"=w5855) -> (w5856:cluster{"Restart flag":u8, "Stage move flag":u8})
                    n600 = local write "Additional Info"(w5856) -> ()
                  }
                  frame True {
                    n601 = stacked-sequence {
                      frame #0 {
                        w5858 = TRUE ("Temperature warning armed")
                        n602 = local read "Last FIB recipe"() -> (w5859:path)
                        n603 = local write "Temperature warning armed"(w5858) -> ()
                        n604 = local write "SW error warning armed"(w5858) -> ()
                        n605 = local write "Focus index warning armed"(w5858) -> ()
                        n606 = local write "Re-engage warning armed"(w5858) -> ()
                        n607 = shared-variable ".\\Zeiss Library.lvlib\\FIB PID reset"(w5858) -> ()  [unwired: 1 in, 1 out]
                        n608 = local write "Read recipe path"(w5859) -> ()
                      }
                      frame #1 {
                        n609 = local write "Load recipe"(TRUE ("Load recipe")) -> ()
                        n610 = local read "Additional Info"() -> (w5863:cluster{"Restart flag":u8, "Stage move flag":u8})
                        n611 = Bundle By Name(cluster=w5863, "Restart flag"=u8 100, "Stage move flag"=u8 0) -> (w5862:cluster{"Restart flag":u8, "Stage move flag":u8})
                        n612 = local write "Additional Info"(w5862) -> ()
                      }
                      frame #2 {
                        n613 = while {
                          stop <- w5865 stop-if-true
                          n614 = local read "Load recipe"() -> (w5869:bool)
                          n615 = Wait Until Next ms Multiple(millisecond multiple=u32 100) -> ()  [unwired: 1 out]
                          n616 = local read "FIB"() -> (w5870:bool)
                          n617 = local read "Stop"() -> (w5866:bool)
                          n618 = Not(x=w5869) -> (.not. x?=w5868:bool)
                          n619 = Not(x=w5870) -> (.not. x?=w5867:bool)
                          n620 = Compound Arithmetic op=OR(w5868, w5867, w5866) -> (w5865:bool)
                        }
                      }
                      frame #3 {
                        n621 = local read "SEM Options"() -> (w5880:T27)
                        n622 = local read "Milling para"() -> (w5898:T35)
                        n623 = shared-variable "My Computer\\Zeiss Library.lvlib\\Milling cont. from Last"(TRUE ("Milling cont. from Last")) -> ()  [unwired: 1 in, 1 out]
                        n624 = local write "Reset Focus"(FALSE ("Reset Focus")) -> ()
                        n625 = local read "Last milling snapshot"() -> (w5895:path)
                        n626 = local read "Last FIB image"() -> (w5907:path)
                        n627 = local read "Last Det A Low Mag"() -> (w5905:path)
                        n628 = local read "Last Det B Low Mag"() -> (w5906:path)
                        n629 = local write "Initial Options"(w5880) -> ()
                        n630 = Bundle By Name(cluster=w5898, "Z offset (um)"=sgl 0.0 ("Y offset (um)")) -> (w5897:T35)
                        n631 = call-poly <vilib>:"Read From XML File.vi"("XML File Path"=w5895) -> ("XML Elements"=w5894:string)  [unwired: 8 in, 2 out]
                        n632 = File/Directory Info(path=w5907) -> (path out=w5909:path, error out=w5910:errorcluster)  [unwired: 1 in, 5 out]
                        n633 = File/Directory Info(path=w5905) -> (path out=w5900:path, error out=w5899:errorcluster)  [unwired: 1 in, 5 out]
                        n634 = File/Directory Info(path=w5906) -> (path out=w5903:path, error out=w5904:errorcluster)  [unwired: 1 in, 5 out]
                        n635 = local write "Milling para"(w5897) -> ()
                        n636 = Unbundle By Name(w5910) -> ("status"=w5908:bool)
                        n637 = Unbundle By Name(w5899) -> ("status"=w5901:bool)
                        n638 = Unbundle By Name(w5904) -> ("status"=w5902:bool)
                        n639 = Unflatten From XML(xml string=w5894, type=T46 {"Timestamp"=timestamp(0 s since 1904-01-01), "Milling Z voltage"=0.0, "FIB slice #"=0, "Pause for reheat"=FALSE, "Last good FI"=0.0, "Focus index"=0.0, "SEM max FOV"=0.0, "Remaining X shift frames"=0, "Remaining Y shift frames"=0} ("output cluster")) -> (value=w5893:T46)  [unwired: 1 in, 1 out]
                        n640 = case shown="False" w5908 {
                          tunnel: w5909 -> [w5926 _]
                          frame False {
                            n641 = call <vilib>:"Read PNG File.vi"("path to PNG file"=w5926) -> ("image data"=w5927:T52)  [unwired: 8 in, 2 out]
                            n642 = call <vilib>:"Unflatten Pixmap.vi"("image data"=w5927) -> ("8-bit pixmap"=w5925:u8[][])  [unwired: 4 in, 6 out]
                            n643 = To Word Integer(number=w5925) -> (16bit integer=w5924:i16[][])
                            n644 = local write "FIB Image"(w5924) -> ()
                            n645 = shared-variable ".\\Zeiss Library.lvlib\\FIB Img"(w5924) -> ()  [unwired: 1 in, 1 out]
                          }
                          frame True {
                          }
                        }
                        n646 = case shown="False" w5901 {
                          tunnel: w5900 -> [w5922 _]
                          frame False {
                            n647 = call <vilib>:"Read PNG File.vi"("path to PNG file"=w5922) -> ("image data"=w5923:T52)  [unwired: 8 in, 2 out]
                            n648 = call <vilib>:"Unflatten Pixmap.vi"("image data"=w5923) -> ("8-bit pixmap"=w5920:u8[][])  [unwired: 4 in, 6 out]
                            n649 = To Word Integer(number=w5920) -> (16bit integer=w5921:i16[][])
                            n650 = local write "Detector A Low Mag"(w5921) -> ()
                          }
                          frame True {
                          }
                        }
                        n651 = case shown="False" w5902 {
                          tunnel: w5903 -> [w5918 _]
                          frame False {
                            n652 = call <vilib>:"Read PNG File.vi"("path to PNG file"=w5918) -> ("image data"=w5919:T52)  [unwired: 8 in, 2 out]
                            n653 = call <vilib>:"Unflatten Pixmap.vi"("image data"=w5919) -> ("8-bit pixmap"=w5917:u8[][])  [unwired: 4 in, 6 out]
                            n654 = To Word Integer(number=w5917) -> (16bit integer=w5916:i16[][])
                            n655 = local write "Detector B Low Mag"(w5916) -> ()
                          }
                          frame True {
                          }
                        }
                        n656 = Unbundle(w5893) -> ("Timestamp"=w5890:timestamp, "Milling Z voltage"=w5892:sgl, "FIB slice #"=w5891:u32, "Pause for reheat"=w5889:bool, "Last good FI"=w5888:sgl, "SEM max FOV"=w5876:sgl, "Remaining X shift frames"=w5873:u32, "Remaining Y shift frames"=w5872:u32)  [unwired: 1 out]
                        "Reheat from last" <- w5889
                        n657 = local read "Hardware Configuration"() -> (w5877:T25)
                        n658 = local write "Remaining X shift frames"(w5873) -> ()
                        n659 = local write "Remaining Y shift frames"(w5872) -> ()
                        n660 = case shown="True" w5889 {
                          tunnel: w5890 -> [_ w5915]
                          tunnel: w5888 -> [_ w5914]
                          frame False {
                            n661 = local write "Pause for reheat"(FALSE ("Reheat")) -> ()
                            n662 = property on="Pause for reheat" class="Bool (strict)"("DisabledEnum"=T44."Enabled" ("Disabled")) -> ()  [unwired: 2 in, 2 out]
                          }
                          frame True {
                            n663 = local write "Pre-reheat time"(w5915) -> ()
                            n664 = local write "Pre-reheat FI"(w5914) -> ()
                            n665 = property on="Pause for reheat" class="Bool (strict)"("DisabledEnum"=T44."Disabled and Grayed Out" ("Disabled")) -> ()  [unwired: 2 in, 2 out]
                          }
                        }
                        n666 = Bundle By Name(cluster=w5877, "SEM Max FOV (um)"=w5876) -> (w5875:T25)
                        n667 = shared-variable ".\\Zeiss Library.lvlib\\Milling Z Voltage Last"(w5892) -> ()  [unwired: 1 in, 1 out]
                        n668 = local write "FIB slice #"(w5891) -> ()
                        n669 = local read "Email Alert Recipients"() -> (w5884:string[])
                        n670 = local write "Hardware Configuration"(w5875) -> ()
